vi "Valid.vi"(11 "EventMessenger in":refnum<class "EventMessenger.lvclass">) -> (2 "Valid?":bool, 3 "EventMessenger out":refnum<class "EventMessenger.lvclass">)   [LabVIEW 2011, in "Messenging.lvlib" / "EventMessenger.lvclass"]
uses:
  EventMessenger.lvclass
  EventMessenger.lvclass/EventMessenger.ctl
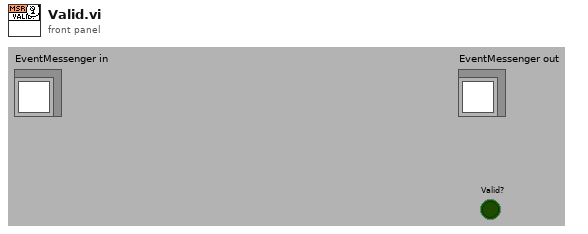
[diagram p1: front panel]
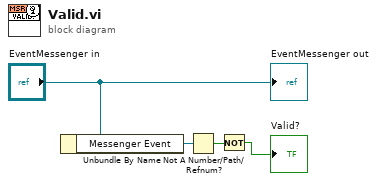
[diagram p0: block diagram]
diagram:
  n1 = Unbundle By Name("EventMessenger in") -> ("Messenger Event"=w3:refnum<user-event>)
  n2 = Not A Number/Path/Refnum?(number/path/refnum=w3) -> (NaN/Path/Refnum?=w2:bool)
  n3 = Not(x=w2) -> (.not. x?=→"Valid?":bool)
  "EventMessenger out" <- "EventMessenger in"
